vi "test_rethinkdb_json.vi"(8 "error in (no error)":errorcluster) -> (0 "error out":errorcluster)   [LabVIEW 2017]
uses:
  rethinkdb/json/rethinkdb_json_token.ctl
panel:
  out "test_case_total":i32
  out "all_passed":bool
  out "test_case":i32
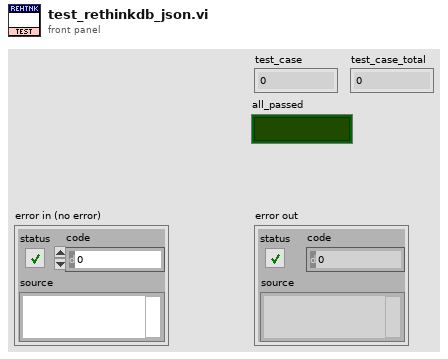
[diagram p1: front panel]
types:
  T1 = typedef "rethinkdb_json_token.ctl" = enum8{"invalid", "null", "boolean", "decimal", "float", "string", "key", "comma", "object_start", "object_end", "array_start", "array_end", "end"}
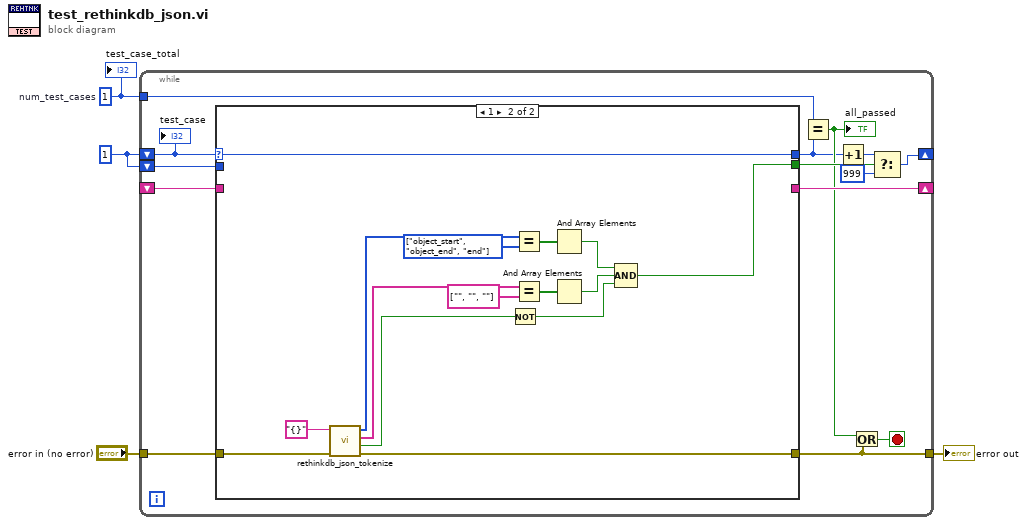
[diagram p0: block diagram]
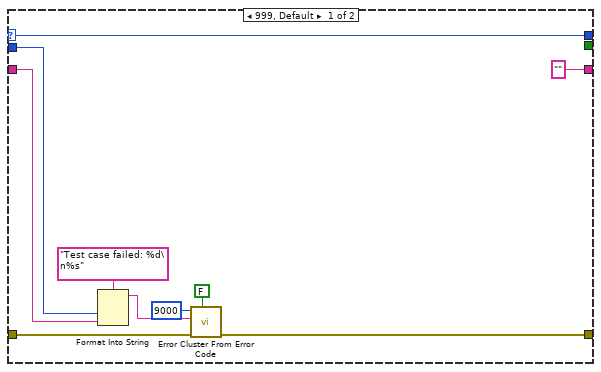
[diagram p2: hidden frame]
diagram:
  w1 = 1  # num_test_cases
  w2 = 1
  n1 = while {
    tunnel: "error in (no error)" -> [w18]
    tunnel: [w7] -> w3
    shift-right: [w10] -> _
    shift-left: w2 -> [w12]
    shift-left: w2 -> [w16]
    shift-right: [w15] -> _
    shift-left: _ -> [w14]
    tunnel: w1 -> [w9]
    stop <- w6 stop-if-true
    n2 = case shown="1" w12 {
      selector: w12 -> [w28 w42]
      tunnel: [w26 w40] -> w7
      tunnel: w18 -> [w27 w41]
      tunnel: [w28 w42] -> w5
      tunnel: w16 -> [w21 _]
      tunnel: ["" _] -> w15
      tunnel: w14 -> [w19 _]
      tunnel: [_ w35] -> w13
      frame 999, Default {
        n3 = Format Into String(format string="Test case failed: %d\n%s" ("error message (\"\")"), w21, w19) -> (resulting string=w22:string)  [unwired: 2 in, 1 out]
        n4 = call <vilib>:"Error Cluster From Error Code.vi"("show call chain? (False)"=FALSE, "error in (no error)"=w27, "error message (\"\")"=w22, "error code (0)"=9000) -> ("error out"=w26:errorcluster)  [unwired: 5 in]
      }
      frame 1 {
        w29 = T1[] [enum."object_start", enum."object_end", enum."end"] items=["invalid", "null", "boolean", "decimal", "float", "string", "key", "comma", "object_start", "object_end", "array_start", "array_end", "end"] ("tokens")
        n5 = call "rethinkdb_json_tokenize.vi"("error in (no error)"=w41, "json"="{}") -> ("error out"=w40:errorcluster, "invalid?"=w39:bool, "args"=w31:string[], "tokens"=w32:T1[])  [unwired: 6 in]
        n6 = Not(x=w39) -> (.not. x?=w36:bool)
        n7 = Equal?(x=w32, y=w29) -> (x = y?=w38:bool[])
        n8 = Equal?(x=w31, y=string[] ["", "", ""] ("args")) -> (x = y?=w37:bool[])
        n9 = And Array Elements(Boolean array=w38) -> (logical AND=w34:bool)
        n10 = And Array Elements(Boolean array=w37) -> (logical AND=w33:bool)
        n11 = Compound Arithmetic op=AND(w34, w33, w36) -> (w35:bool)
      }
    }
    n12 = Equal?(x=w9, y=w5) -> (x = y?=w8:bool)
    "all_passed" <- w8
    n13 = Increment(x=w5) -> (x+1=w11:i32)
    n14 = Or(x=w8, y=w7) -> (x .or. y?=w6:bool)
    n15 = Select(t=w11, s=w13, f=999) -> (s? t:f=w10:i32)
    "test_case" <- w12
  }
  "error out" <- w3
  "test_case_total" <- w1
